vi "FT10_M4X Tester.vi"() -> ()   [LabVIEW 2024]
uses:
  Controls/QMH Fundamentals - Message Cluster.ctl
  <vilib>/FPGAPlugInAG/PXI-7854R/niLvFpga_Open_PXI-7854R.vi
  <vilib>/rvi/interface/common/dynamic/niFpgaDynamicAddResources.vi
  <vilib>/Utility/error.llb/Error Cluster From Error Code.vi
  <vilib>/rvi/errors/niLvFpgaAdjustHostInterfaceError.vi
  <vilib>/FPGAPlugInAG/Dynamic/niLvFpga_Close_Dynamic.vi
  <vilib>/rvi/interface/nirviOpenFPGA/nirviOpenFPGA.xnode
  FPGA Bitfiles/7_11_2024_FT10_FPGA_7854R_Main_Rev2 BitFile.lvbitx
  <vilib>/rvi/interface/nirviReadWriteControl/nirviReadWriteControl.xnode
  <vilib>/rvi/interface/nirviCloseFPGA/nirviCloseFPGA.xnode
  spcm_win32.dll
  NiFpgaLv.dll
  <vilib>/rvi/interface/Simulation/niFpgaSimulationCallBeginRW.vi
panel:
  out "error out 2":errorcluster
  in  "Conn2/DIO_16_23 In":bool[](array[boolean])=[FALSE, FALSE, FALSE, FALSE, FALSE, FALSE, FALSE, FALSE]
  out "Conn2/DIO_16_23 Out":bool[](array[boolean])
  out "Conn2/DIO_8_15 Out":bool[](array[boolean])
  out "Conn2/DIO_0_7 Out":bool[](array[boolean])
  in  "Conn2/DIO_8_15 In":bool[](array[boolean])=[FALSE, FALSE, FALSE, FALSE, FALSE, FALSE, FALSE, FALSE]
  in  "Conn2/DIO_0_7 In":bool[](array[boolean])=[FALSE, FALSE, FALSE, FALSE, FALSE, FALSE, FALSE, FALSE]
  in  "75kHz":bool=TRUE
  in  "uSec Off":u16=6
  in  "uSec On":u16=7
  in  "Update Relays":bool
  in  "index 2":i32=2
  in  "index":i32
  out "Waveform Array":waveform(dbl)[](graph)
  out "appended array":waveform(dbl)[](array[waveform])
  out "Array":T1(array[cluster])
  in  "stop":bool
  in  "Read":bool
  out "error out":errorcluster
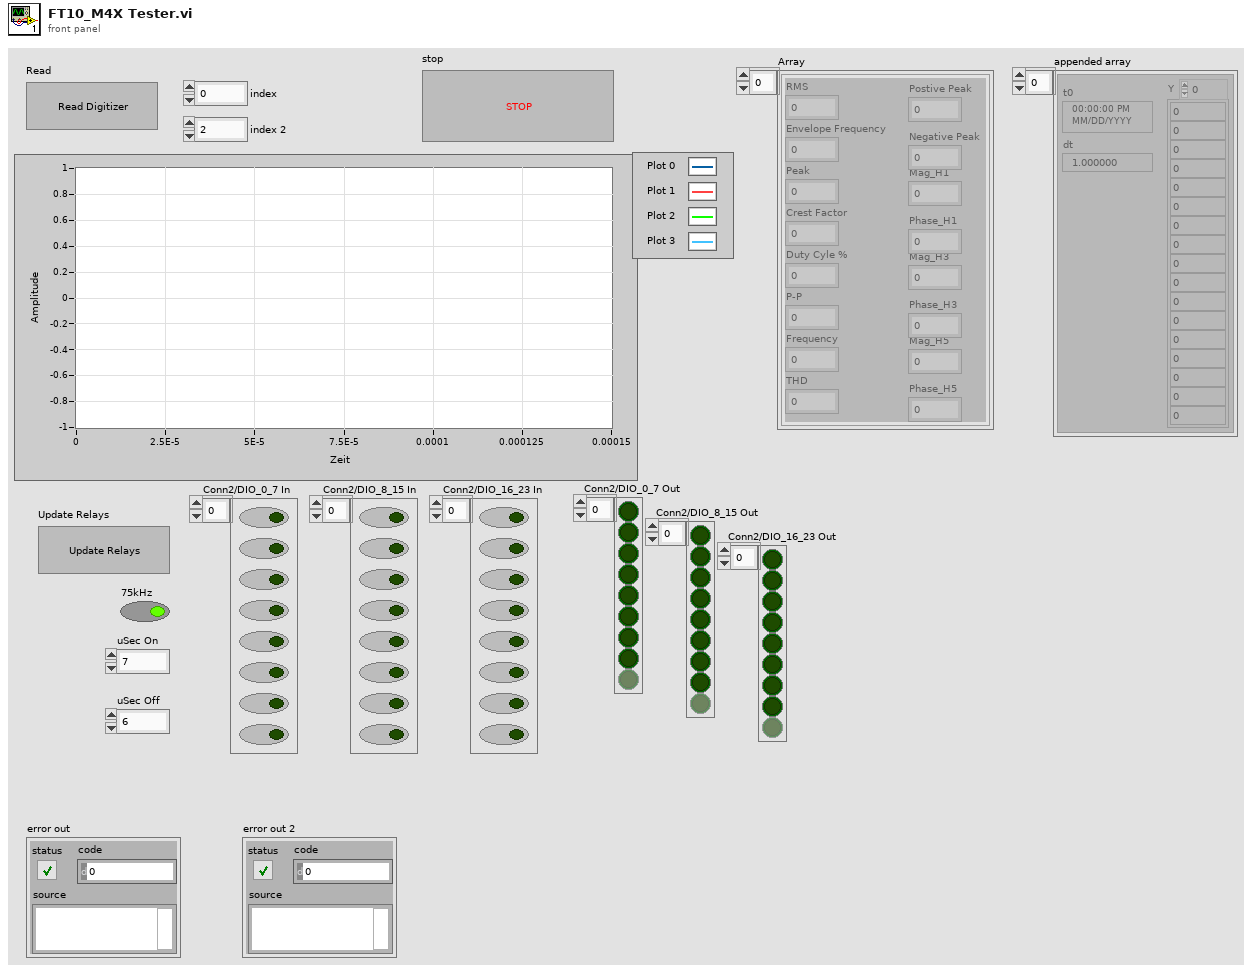
[diagram p1: front panel]
types:
  T1 = cluster{"RMS":dbl, "Envelope Frequency":dbl, "Peak":dbl, "Crest Factor":dbl, "Duty Cyle %":dbl, "P-P":dbl, "Frequency":dbl, "THD":dbl, "Postive Peak":dbl, "Negative Peak":dbl, "Mag_H1":dbl, "Phase_H1":dbl, "Mag_H3":dbl, "Phase_H3":dbl, "Mag_H5":dbl, "Phase_H5":dbl}[]
  T2 = typedef "QMH Fundamentals - Message Cluster.ctl" = cluster{"Message":string, "Message Data":variant}
  T3 = cluster{"RMS":dbl, "Envelope Frequency":dbl, "Peak":dbl, "Crest Factor":dbl, "Duty Cyle %":dbl, "P-P":dbl, "Frequency":dbl, "THD":dbl, "Postive Peak":dbl, "Negative Peak":dbl, "Mag_H1":dbl, "Phase_H1":dbl, "Mag_H3":dbl, "Phase_H3":dbl, "Mag_H5":dbl, "Phase_H5":dbl}
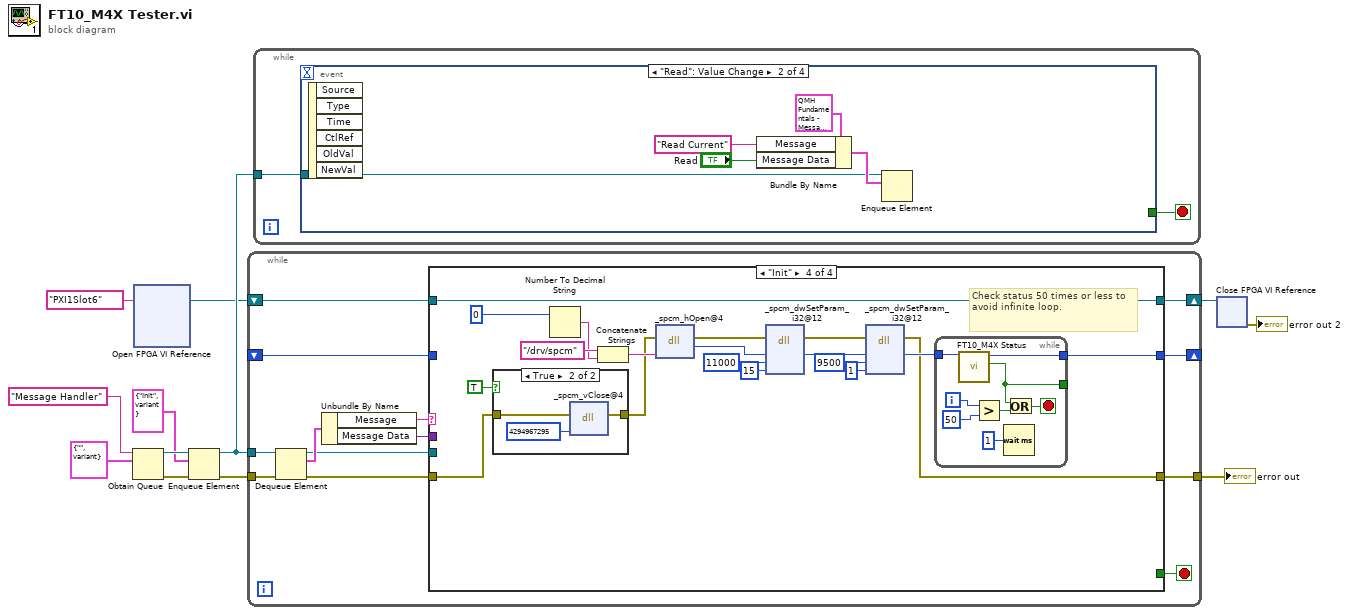
[diagram p0: block diagram]
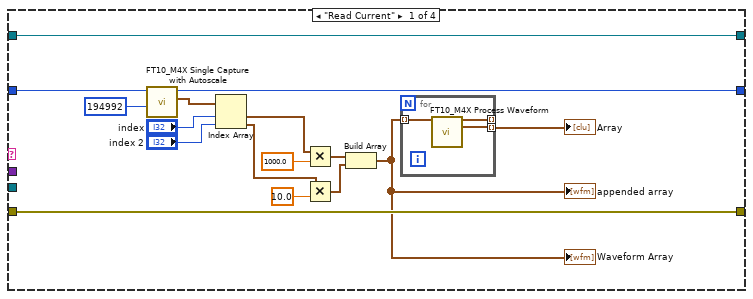
[diagram p2: hidden frame]
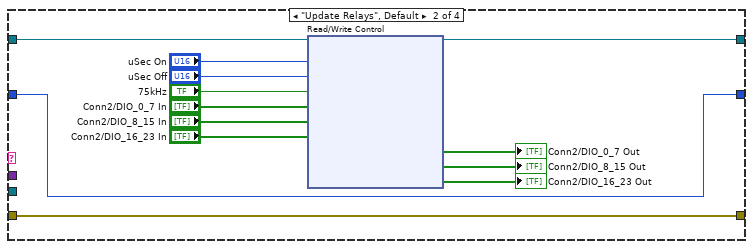
[diagram p3: hidden frame]
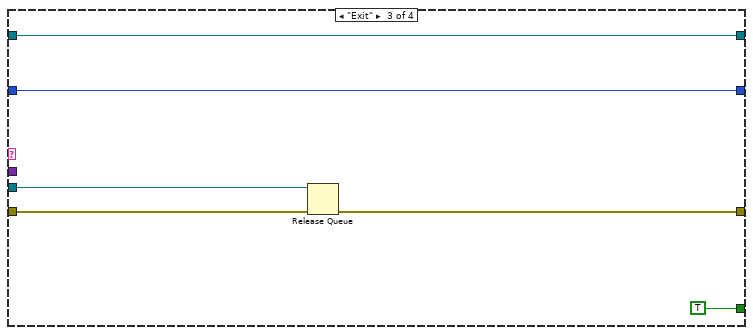
[diagram p4: hidden frame]
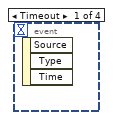
[diagram p6: hidden frame]
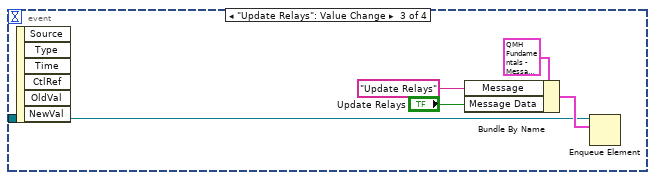
[diagram p7: hidden frame]
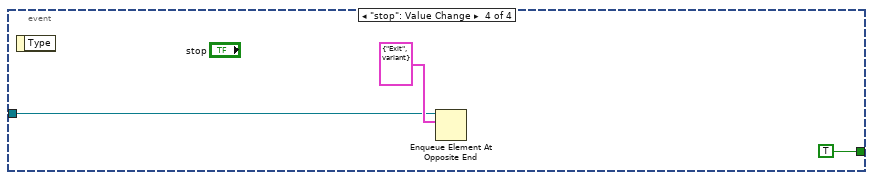
[diagram p8: hidden frame]
diagram:
  n1 = Obtain Queue(name (unnamed)="Message Handler", element data type=T2 {"Message"="", "Message Data"=variant} ("Message Cluster")) -> (queue out=w10:refnum<queue>, error out=w11:errorcluster)  [unwired: 3 in, 1 out]
  n2 = xnode "Open FPGA VI Reference"("resource name"=tag "PXI1Slot6") -> ("FPGA VI Reference Out"=w3:refnum<k20>)  [unwired: 1 in, 1 out]
  n3 = Enqueue Element(queue=w10, element=T2 {"Message"="Init", "Message Data"=variant}, error in (no error)=w11) -> (queue out=w5:refnum<queue>, error out=w7:errorcluster)  [unwired: 1 in, 1 out]
  n4 = while {
    tunnel: w5 -> [w24]
    tunnel: w7 -> [w23]
    tunnel: [w18] -> w6
    shift-right: [w17] -> _
    shift-left: _ -> [w16]
    shift-right: [w14] -> w2
    shift-left: w3 -> [w13]
    stop <- w15 stop-if-true
    n5 = Dequeue Element(queue=w24, error in (no error)=w23) -> (queue out=w22:refnum<queue>, element=w25:T2, error out=w21:errorcluster)  [unwired: 1 in, 1 out]
    n6 = Unbundle By Name(w25) -> ("Message"=w20:string, "Message Data"=w19:variant)
    n7 = case shown="\"Init\"" w20 {
      tunnel: w22 -> [_ _ w59 _]
      tunnel: w21 -> [w30 w45 w61 w67]
      tunnel: w19 -> [_ _ _ _]
      tunnel: [w30 w45 w60 w66] -> w18
      tunnel: [w31 w46 w63 w65] -> w17
      tunnel: w16 -> [w32 w46 w63 _]
      tunnel: [_ _ TRUE _] -> w15
      tunnel: [w26 w47 w58 w64] -> w14
      tunnel: w13 -> [w26 w48 w58 w64]
      frame "Read Current" {
        n8 = call "FT10_M4X Single Capture with Autoscale.vi"("memsize"=194992, "Card Handle in"=w32) -> ("Data"=w35:waveform(sgl)[], "Card Handle out"=w31:u32)  [unwired: 8 in]
        n9 = Index Array(array=w35, index #1="index", index #2="index 2") -> (element #1=w40:waveform(sgl), element #2=w41:waveform(sgl))
        n10 = Multiply(x=w40, y=1000.0) -> (x*y=w38:waveform(dbl))
        n11 = Multiply(x=w41, y=10.0) -> (x*y=w39:waveform(dbl))
        n12 = Build Array(w38, w39) -> (w29:waveform(dbl)[])
        "appended array" <- w29
        "Waveform Array" <- w29
        n13 = for {
          tunnel: w29 -> [w42] mode=indexing
          tunnel: [w44] -> w33 mode=indexing
          tunnel: [w43] -> _ mode=indexing
          n14 = call "FT10_M4X Process Waveform.vi"("RF Waveform In"=w42) -> ("RF Waveform Out"=w43:waveform(sgl), "Measurements"=w44:T3)  [unwired: 12 in, 1 out]
        }
        "Array" <- w33
      }
      frame "Update Relays", Default {
        n15 = xnode "Read/Write Control"("FPGA VI Reference In"=w48, "uSec On"="uSec On", "uSec Off"="uSec Off", "75kHz"="75kHz", "Conn2/DIO_0_7 In"="Conn2/DIO_0_7 In", "Conn2/DIO_8_15 In"="Conn2/DIO_8_15 In", "Conn2/DIO_16_23 In"="Conn2/DIO_16_23 In") -> ("FPGA VI Reference Out"=w47:refnum<k20>, "Conn2/DIO_0_7 Out"=→"Conn2/DIO_0_7 Out":bool[], "Conn2/DIO_8_15 Out"=→"Conn2/DIO_8_15 Out":bool[], "Conn2/DIO_16_23 Out"=→"Conn2/DIO_16_23 Out":bool[])  [unwired: 1 in, 1 out]
      }
      frame "Exit" {
        n16 = Release Queue(queue=w59, error in (no error)=w61) -> (error out=w60:errorcluster)  [unwired: 1 in, 2 out]
      }
      frame "Init" {
        # "Check status 50 times or less to avoid infinite loop."
        n17 = case shown="True" TRUE ("reset device") {
          tunnel: w67 -> [w91 w94]
          tunnel: [w91 w93] -> w77
          frame False {
          }
          frame True {
            n18 = dll-call lib="spcm_win32.dll" fn="_spcm_vClose@4"(error in=w94, "hDrv"=u32 4294967295) -> (error out=w93:errorcluster)  [unwired: 4 in, 1 out]
          }
        }
        n19 = Number To Decimal String(number=u32 0 ("Board #")) -> (decimal integer string=w78:string)  [unwired: 1 in]
        n20 = Concatenate Strings("/drv/spcm" ("szDeviceName"), w78) -> (w79:string)
        n21 = dll-call lib="spcm_win32.dll" fn="_spcm_hOpen@4"(error in=w77, "szDeviceName"=w79) -> (error out=w75:errorcluster, "hDrv"=w74:u32)  [unwired: 3 in, 1 out]
        n22 = dll-call lib="spcm_win32.dll" fn="_spcm_dwSetParam_i32@12" label="SPC_CHENABLE"(error in=w75, "hDrv"=w74, "lRegister"=11000, "lValue"=15) -> (error out=w71:errorcluster, "hDrv"=w70:u32)  [unwired: 5 in, 1 out]
        n23 = dll-call lib="spcm_win32.dll" fn="_spcm_dwSetParam_i32@12" label="SPC_CARDMODE"(error in=w71, "hDrv"=w70, "lRegister"=9500, "lValue"=1) -> (error out=w66:errorcluster, "hDrv"=w82:u32)  [unwired: 5 in, 1 out]
        n24 = while {
          tunnel: w82 -> [w89]
          tunnel: [w88] -> w65
          tunnel: [w83] -> _
          i -> [w87]
          stop <- w85 stop-if-true
          n25 = call "FT10_M4X Status.vi"("Card Handle in"=w89) -> ("Ready?"=w83:bool, "Card Handle out"=w88:u32)  [unwired: 9 in]
          n26 = Greater?(x=w87, y=50) -> (0:w84:bool)
          n27 = Wait (ms)(milliseconds to wait=u32 1) -> ()  [unwired: 1 out]
          n28 = Or(x=w83, y=w84) -> (x .or. y?=w85:bool)
        }
      }
    }
  }
  "error out" <- w6
  n29 = while {
    tunnel: w5 -> [w96]
    stop <- w95 stop-if-true
    n30 = event shown="[1] \"Read\": Value Change" {
      selector: _ -> [_ _ _ _]
      dyn-events: _ -> [_ _ _ _]
      timeout: _ -> [_ _ _ _]
      tunnel: w96 -> [_ w98 w103 w108]
      tunnel: [_ _ _ TRUE] -> w95
      event Timeout {
        n31 = event-data() -> ()  [unwired: 1 in, 3 out]
      }
      event "Read": Value Change {
        n32 = event-data() -> ()  [unwired: 1 in, 6 out]
        n33 = Bundle By Name(cluster=T2 {"Message"="Fornax Connect/Disconnect", "Message Data"=variant} ("element"), "Message"="Read Current", "Message Data"="Read") -> (w99:T2)
        n34 = Enqueue Element(queue=w98, element=w99) -> ()  [unwired: 2 in, 3 out]
      }
      event "Update Relays": Value Change {
        n35 = event-data() -> ()  [unwired: 1 in, 6 out]
        n36 = Bundle By Name(cluster=T2 {"Message"="Fornax Connect/Disconnect", "Message Data"=variant} ("element"), "Message"="Update Relays", "Message Data"="Update Relays") -> (w104:T2)
        n37 = Enqueue Element(queue=w103, element=w104) -> ()  [unwired: 2 in, 3 out]
      }
      event "stop": Value Change {
        n38 = event-data() -> ()  [unwired: 1 in, 1 out]
        n39 = Enqueue Element At Opposite End(queue=w108, element=T2 {"Message"="Exit", "Message Data"=variant}) -> ()  [unwired: 2 in, 3 out]
      }
    }
  }
  n40 = xnode "Close FPGA VI Reference"("FPGA VI Reference In"=w2) -> ("error out"=→"error out 2":errorcluster)  [unwired: 1 in]
